vi "Calc Text Width.vi"(11 "State":T1) -> (2 "Value Width":i16, 3 "Name Width":i16, 5 "Name Center":i16, 7 "Min Width":i16)   [LabVIEW 2020, in "Parallel Diagram Block.xnode"]
uses:
  Parallel Diagram Block.xnode
  State.ctl
  Parallel Block/Type Descriptor.ctl
  Parallel Block/Direction.ctl
  Parallel Block/Value Type.ctl
  Parallel Block/Terminal Mode.ctl
  Parallel Block/Terminal Type.ctl
  Parallel Block/Type Mode.ctl
  Parallel Block/Value Mode.ctl
  <vilib>/picture/picture.llb/imagedata.ctl
  Parallel Block/Manager Node.ctl
  Parallel Block/Parallel Block.lvlib
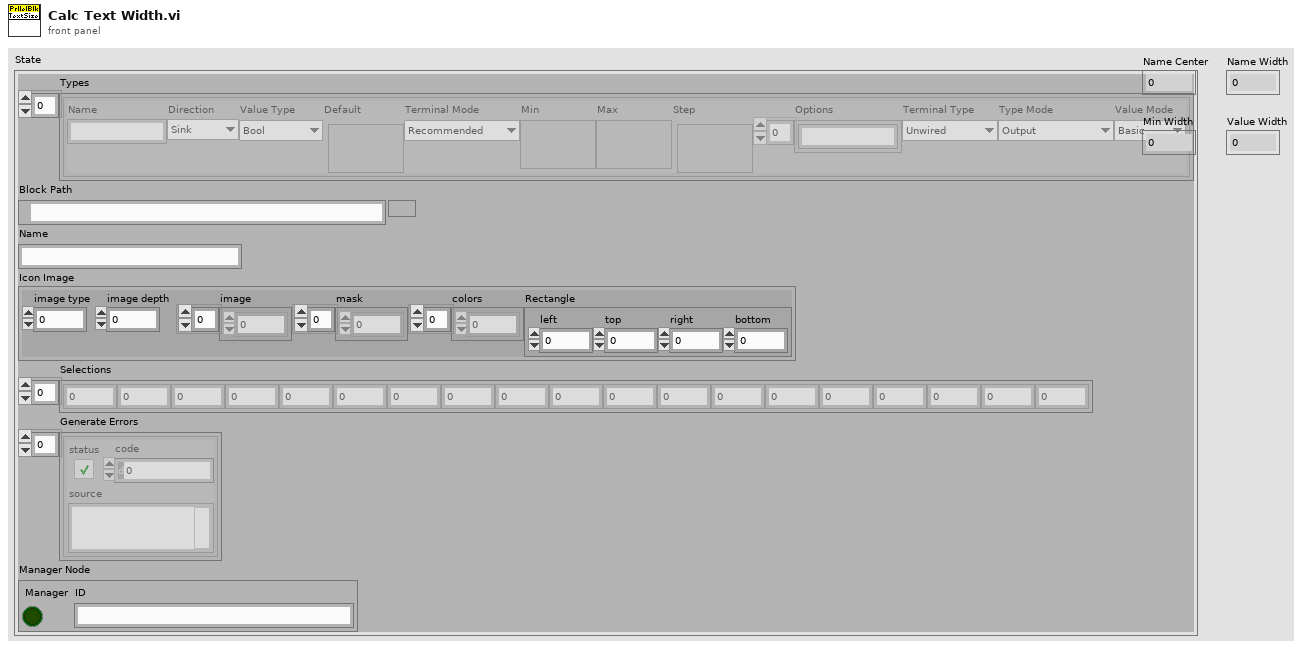
[diagram p1: front panel]
types:
  T1 = typedef "Parallel Diagram Block.xnode/State.ctl" = cluster{"Types":T2[], "Block Path":path, "Name":string, "Icon Image":T9, "Selections":i32[], "Generate Errors":errorcluster[], "Manager Node":T10}
  T2 = typedef "Parallel Block.lvlib/Type Descriptor.ctl" = cluster{"Name":string, "Direction":T3, "Value Type":T4, "Default":variant, "Terminal Mode":T5, "Min":variant, "Max":variant, "Step":variant, "Options":string[], "Terminal Type":T6, "Type Mode":T7, "Value Mode":T8}
  T3 = typedef "Parallel Block.lvlib/Direction.ctl" = enum16{"Sink", "Source"}
  T4 = typedef "Parallel Block.lvlib/Value Type.ctl" = enum16{"Unknown", "Bool", "U8", "U16", "U32", "U64", "I8", "I16", "I32", "I64", "SGL", "DBL", "CSG", "CDB", "CDBWfm", "String", "DBLWfm"}
  T5 = typedef "Parallel Block.lvlib/Terminal Mode.ctl" = enum16{"Recommended", "Required", "None"}
  T6 = typedef "Parallel Block.lvlib/Terminal Type.ctl" = enum16{"Unwired", "BadType", "Connection", "Value", "Control Ref", "BadRefType"}
  T7 = typedef "Parallel Block.lvlib/Type Mode.ctl" = enum16{"Output", "Single - Strict", "Single - Coerced", "Stream"}
  T8 = typedef "Parallel Block.lvlib/Value Mode.ctl" = enum16{"Basic", "Range", "Select"}
  T9 = typedef "imagedata.ctl" = cluster{"image type":i32, "image depth":i32, "image":u8[], "mask":u8[], "colors":u32[], "Rectangle":cluster{"left":i16, "top":i16, "right":i16, "bottom":i16}}
  T10 = typedef "Parallel Block.lvlib/Manager Node.ctl" = cluster{"Manager":bool, "ID":string}
  T11 = cluster{"left":i16, "top":i16, "right":i16, "bottom":i16}
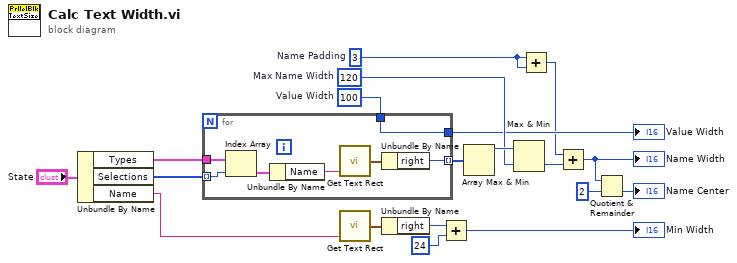
[diagram p0: block diagram]
diagram:
  w9 = i16 100  # Value Width
  w1 = i16 3  # Name Padding
  w14 = i16 120  # Max Name Width
  n1 = Unbundle By Name("State") -> ("Types"=w18:T2[], "Selections"=w17:i32[], "Name"=w7:string)
  n2 = for {
    tunnel: w18 -> [w26]
    tunnel: w17 -> [w25] mode=indexing
    tunnel: [w21] -> w16 mode=indexing
    tunnel: w9 -> [w20]
    tunnel: [w20] -> w8
    n3 = Index Array(array=w26, index=w25) -> (element=w24:T2)
    n4 = Unbundle By Name(w24) -> ("Name"=w23:string)
    n5 = call <vilib>:"Get Text Rect.vi"("text"=w23) -> ("rect"=w22:T11)  [unwired: 8 in]
    n6 = Unbundle By Name(w22) -> ("right"=w21:i16)
  }
  "Value Width" <- w8
  n7 = call <vilib>:"Get Text Rect.vi"("text"=w7) -> ("rect"=w6:T11)  [unwired: 8 in]
  n8 = Unbundle By Name(w6) -> ("right"=w5:i16)
  n9 = Add(x=w5, y=i16 24) -> (x+y=→"Min Width":i16)
  n10 = Array Max & Min(array=w16) -> (max value=w15:i16)  [unwired: 3 out]
  n11 = Max & Min(x=w15, y=w14) -> (min(x,y)=w13:i16)  [unwired: 1 out]
  n12 = Add(x=w1, y=w1) -> (x+y=w2:i16)
  n13 = Add(x=w2, y=w13) -> (x+y=w10:i16)
  "Name Width" <- w10
  n14 = Quotient & Remainder(x=w10, y=i16 2) -> (floor(x/y)=→"Name Center":i16)  [unwired: 1 out]
